vi "GuiderControl.vi"() -> ()   [LabVIEW 2011]
panel:
  out "Error":bool
  in  "Filter Position":u16(ring) items=["1"=1, "2"=2, "3"=3, "4"=4, "5"=5, "6"=6]
  in  "Initialize":bool
  in  "Close":bool
  in  "Move Focus":bool
  in  "Relative Focus Steps":i32(slide) min=-5000 max=5000 step=10 scale=-500.0..500.0
  # "Guider Filters\n\t1\t\tEmpty (default)\n\t2\t\tRed      \n\t3\t\tNeutral \t  5\t\tGreen\n\t4\t\tEmpty      6\t\tBlue"
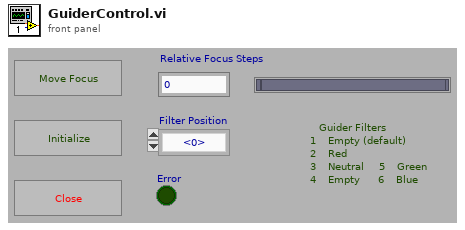
[diagram p1: front panel]
types:
  T1 = enum32{"invalid app kind", "Development System", "Run Time System", "Student Edition", "Embedded LabVIEW", "Evaluation", "Custom"}
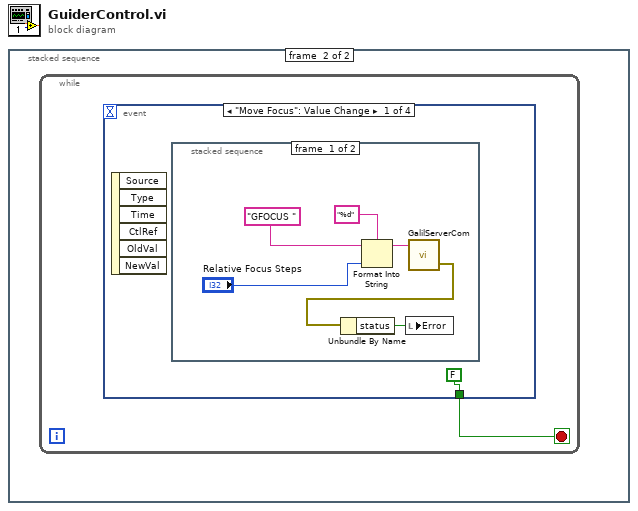
[diagram p0: block diagram]
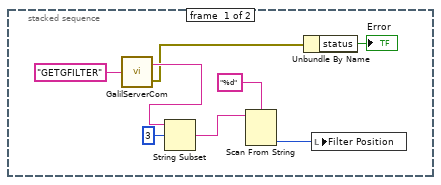
[diagram p2: hidden frame]
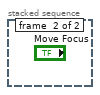
[diagram p3: hidden frame]
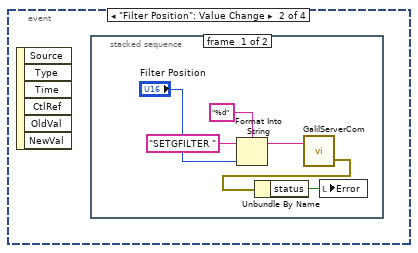
[diagram p4: hidden frame]
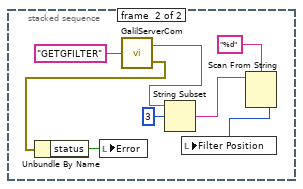
[diagram p5: hidden frame]
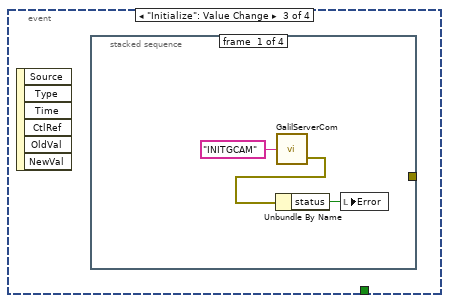
[diagram p6: hidden frame]
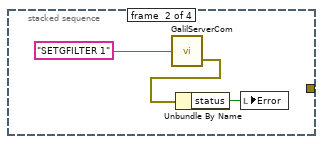
[diagram p7: hidden frame]
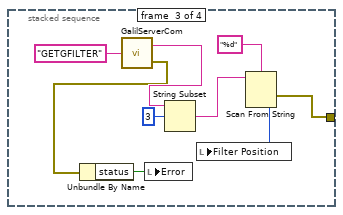
[diagram p8: hidden frame]
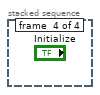
[diagram p9: hidden frame]
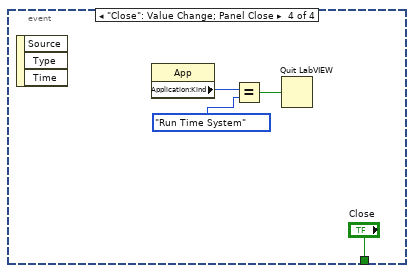
[diagram p10: hidden frame]
diagram:
  n1 = stacked-sequence {
    frame #0 {
      n2 = call "GalilServerCom.vi"("Input"="GETGFILTER") -> ("Output"=w6:string, "error out"=w2:errorcluster)
      n3 = String Subset(string=w6, offset (0)=3) -> (substring=w4:string)  [unwired: 1 in]
      n4 = Scan From String(format string="%d", input string=w4) -> (output 1=w3:i32)  [unwired: 3 in, 3 out]
      n5 = Unbundle By Name(w2) -> ("status"=→"Error":bool)
      n6 = local write "Filter Position"(w3) -> ()
    }
    frame #1 {
      n7 = while {
        stop <- w9 stop-if-true
        n8 = event shown="[0] \"Move Focus\": Value Change" {
          selector: _ -> [_ _ _ _]
          dyn-events: _ -> [_ _ _ _]
          timeout: _ -> [_ _ _ _]
          tunnel: [FALSE ("Quit") _ _ "Close"] -> w9
          event "Move Focus": Value Change {
            n9 = event-data() -> ()  [unwired: 1 in, 6 out]
            n10 = stacked-sequence {
              frame #0 {
                n11 = Format Into String(format string="%d", initial string="GFOCUS " ("Input"), "Relative Focus Steps") -> (resulting string=w14:string)  [unwired: 1 in, 1 out]
                n12 = call "GalilServerCom.vi"("Input"=w14) -> ("error out"=w11:errorcluster)  [unwired: 1 out]
                n13 = Unbundle By Name(w11) -> ("status"=w12:bool)
                n14 = local write "Error"(w12) -> ()
              }
              frame #1 {
              }
            }
          }
          event "Filter Position": Value Change {
            n15 = event-data() -> ()  [unwired: 1 in, 6 out]
            n16 = stacked-sequence {
              frame #0 {
                n17 = Format Into String(format string="%d", initial string="SETGFILTER ", "Filter Position") -> (resulting string=w19:string)  [unwired: 1 in, 1 out]
                n18 = call "GalilServerCom.vi"("Input"=w19) -> ("error out"=w17:errorcluster)  [unwired: 1 out]
                n19 = Unbundle By Name(w17) -> ("status"=w18:bool)
                n20 = local write "Error"(w18) -> ()
              }
              frame #1 {
                n21 = call "GalilServerCom.vi"("Input"="GETGFILTER") -> ("Output"=w28:string, "error out"=w23:errorcluster)
                n22 = Unbundle By Name(w23) -> ("status"=w24:bool)
                n23 = local write "Error"(w24) -> ()
                n24 = String Subset(string=w28, offset (0)=3) -> (substring=w26:string)  [unwired: 1 in]
                n25 = Scan From String(format string="%d", input string=w26) -> (output 1=w25:i32)  [unwired: 3 in, 3 out]
                n26 = local write "Filter Position"(w25) -> ()
              }
            }
          }
          event "Initialize": Value Change {
            n27 = event-data() -> ()  [unwired: 1 in, 6 out]
            n28 = stacked-sequence {
              tunnel: [_ _ w39 _] -> _
              frame #0 {
                n29 = call "GalilServerCom.vi"("Input"="INITGCAM") -> ("error out"=w31:errorcluster)  [unwired: 1 out]
                n30 = Unbundle By Name(w31) -> ("status"=w32:bool)
                n31 = local write "Error"(w32) -> ()
              }
              frame #1 {
                n32 = call "GalilServerCom.vi"("Input"="SETGFILTER 1" ("initial string")) -> ("error out"=w34:errorcluster)  [unwired: 1 out]
                n33 = Unbundle By Name(w34) -> ("status"=w35:bool)
                n34 = local write "Error"(w35) -> ()
              }
              frame #2 {
                n35 = call "GalilServerCom.vi"("Input"="GETGFILTER") -> ("Output"=w43:string, "error out"=w37:errorcluster)
                n36 = Unbundle By Name(w37) -> ("status"=w38:bool)
                n37 = local write "Error"(w38) -> ()
                n38 = String Subset(string=w43, offset (0)=3) -> (substring=w41:string)  [unwired: 1 in]
                n39 = Scan From String(format string="%d", input string=w41) -> (error out=w39:errorcluster, output 1=w40:i32)  [unwired: 3 in, 2 out]
                n40 = local write "Filter Position"(w40) -> ()
              }
              frame #3 {
              }
            }
          }
          event "Close": Value Change; Panel Close {
            n41 = event-data() -> ()  [unwired: 1 in, 3 out]
            n42 = property class="App"() -> ("Application:Kind"=w46:T1)  [unwired: 2 in, 2 out]
            n43 = Equal?(x=w46, y=T1."Run Time System" ("Application:Kind")) -> (x = y?=w48:bool)
            n44 = Quit LabVIEW(quit? (T)=w48) -> ()
          }
        }
      }
    }
  }
